vi "Queue Event Log.vi"(5 "System Data":T1 {"Converter Faults 2" format="%016b"; "Converter Alarms 2" format="%016b"; "Converter Faults 1" format="%016b"; "Converter Alarms 1" format="%016b"; "Solar Faults" format="%016b"; "ES Rack 10 Alarms" format="%016b"; "ES Rack 9 Alarms" format="%016b"; "ES Rack 8 Alarms" format="%016b"; "ES Rack 7 Alarms" format="%016b"; "ES Rack 6 Alarms" format="%016b"; "ES Rack 5 Alarms" format="%016b"; "ES Rack 4 Alarms" format="%016b"; "ES Rack 3 Alarms" format="%016b"; "ES Rack 2 Alarms" format="%016b"; "ES Rack 1 Alarms" format="%016b"; "ES System Alarms" format="%016b"; "System Faults" format="%016b"; "ES Rack 10 Faults" format="%016b"; "Es Rack 9 Faults" format="%016b"; "ES Rack 8 Faults" format="%016b"; "ES Rack 7 Faults" format="%016b"; "ES Rack 6 Faults" format="%016b"; "ES Rack 5 Faults" format="%016b"; "ES Rack 4 Faults" format="%016b"; "ES Rack 3 Faults" format="%016b"; "ES Rack 2 Faults" format="%016b"; "ES Rack 1 Faults" format="%016b"; "ES System Faults" format="%016b"; "System Status" format="%016b"; "Controller Faults" format="%016b"}, 7 "Connection Error":bool, 8 "Error In":errorcluster, 11 "Event Log Queue":refnum<queue>) -> (0 "Error Out":errorcluster)   [LabVIEW 2014]
uses:
  Controls/Modbus Status Interface Data MOD2.ctl
panel:
  in  "Gen East Faults":string
  in  "Gen West Faults":string
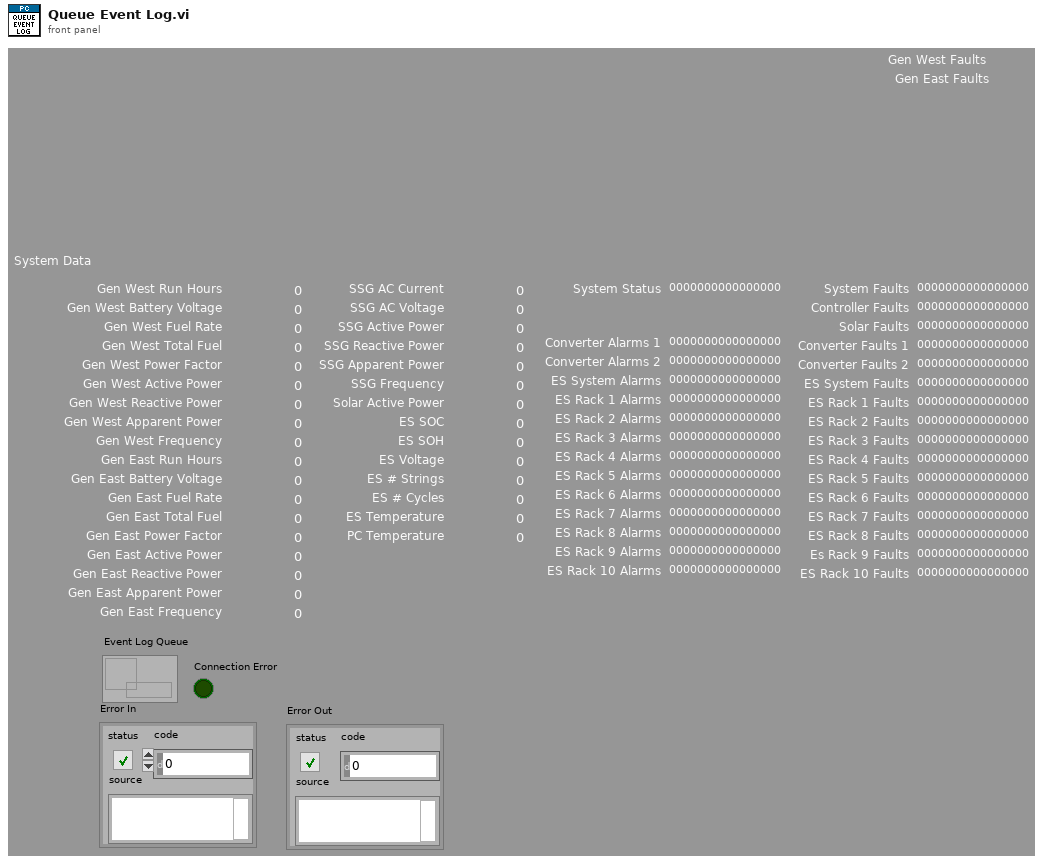
[diagram p1: front panel]
types:
  T1 = typedef "Modbus Status Interface Data MOD2.ctl" = cluster{"SSG AC Current":i16, "SSG AC Voltage":i16, "SSG Active Power":i16, "SSG Reactive Power":i16, "SSG Apparent Power":i16, "SSG Frequency":i16, "ES SOC":i16, "ES SOH":i16, "ES Voltage":i16, "ES # Strings":i16, "ES # Cycles":i16, "ES Temperature":i16, "PC Temperature":i16, "Solar Active Power":i16, "Gen West Run Hours":i16, "Gen West Battery Voltage":i16, "Gen West Fuel Rate":i16, "Gen West Total Fuel":i16, "Gen West Power Factor":i16, "Gen West Active Power":i16, "Gen West Reactive Power":i16, "Gen West Apparent Power":i16, "Gen West Frequency":i16, "Gen East Run Hours":i16, "Gen East Battery Voltage":i16, "Gen East Fuel Rate":i16, "Gen East Total Fuel":i16, "Gen East Power Factor":i16, "Gen East Active Power":i16, "Gen East Reactive Power":i16, "Gen East Apparent Power":i16, "Gen East Frequency":i16, "Converter Version":i16, "Controller Version":i16, "System Status":i16, "System Faults":i16, "Controller Faults":i16, "ES System Faults":i16, "ES System Alarms":i16, "Converter Faults 1":i16, "Converter Faults 2":i16, "Converter Alarms 1":i16, "Converter Alarms 2":i16, "Solar Faults":i16, "ES Rack 1 Faults":i16, "ES Rack 2 Faults":i16, "ES Rack 3 Faults":i16, "ES Rack 4 Faults":i16, "ES Rack 5 Faults":i16, "ES Rack 6 Faults":i16, "ES Rack 7 Faults":i16, "ES Rack 8 Faults":i16, "Es Rack 9 Faults":i16, "ES Rack 10 Faults":i16, "ES Rack 1 Alarms":i16, "ES Rack 2 Alarms":i16, "ES Rack 3 Alarms":i16, "ES Rack 4 Alarms":i16, "ES Rack 5 Alarms":i16, "ES Rack 6 Alarms":i16, "ES Rack 7 Alarms":i16, "ES Rack 8 Alarms":i16, "ES Rack 9 Alarms":i16, "ES Rack 10 Alarms":i16}
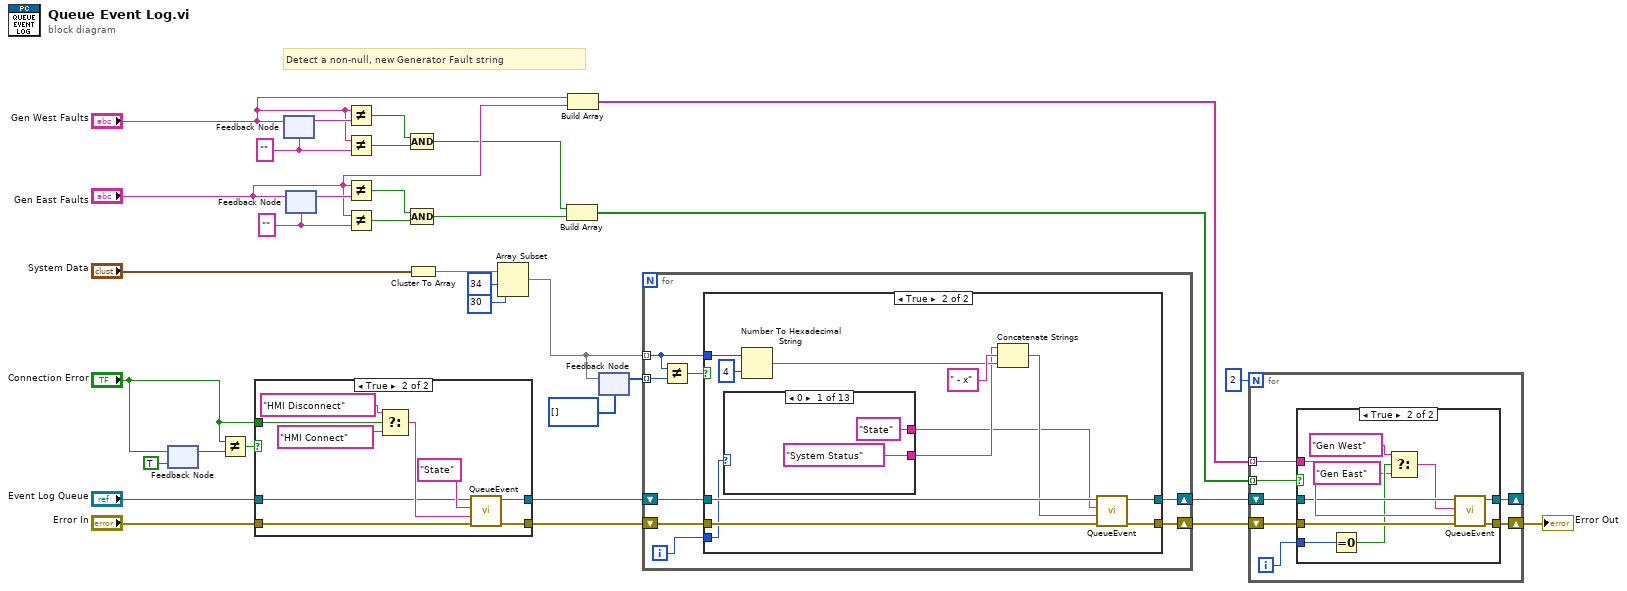
[diagram p0: block diagram]
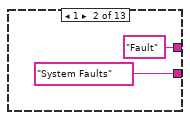
[diagram p4: hidden frame]
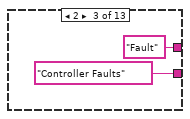
[diagram p5: hidden frame]
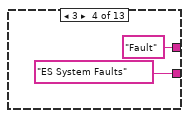
[diagram p6: hidden frame]
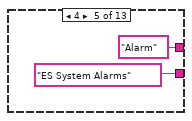
[diagram p7: hidden frame]
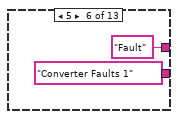
[diagram p8: hidden frame]
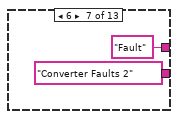
[diagram p9: hidden frame]
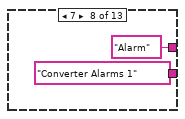
[diagram p10: hidden frame]
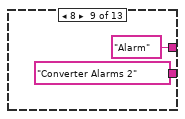
[diagram p11: hidden frame]
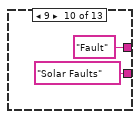
[diagram p12: hidden frame]
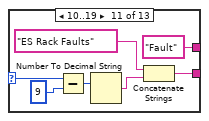
[diagram p13: hidden frame]
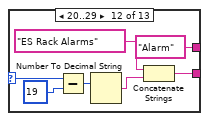
[diagram p14: hidden frame]
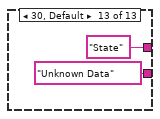
[diagram p15: hidden frame]
diagram:
  w9 = "" ("Gen West Faults")
  w7 = "" ("Gen West Faults")
  # "Detect a non-null, new Generator Fault string"
  n1 = feedback-in #1("Connection Error") -> ()
  n2 = feedback #1(TRUE ("Connection Error")) -> (w30:bool)
  n3 = Not Equal?(x="Connection Error", y=w30) -> (x != y?=w29:bool)
  n4 = case shown="True" w29 {
    tunnel: "Error In" -> [w35 w44]
    tunnel: [w35 w43] -> w22
    tunnel: "Event Log Queue" -> [w34 w38]
    tunnel: "Connection Error" -> [_ w37]
    tunnel: [w34 w36] -> w23
    frame False {
    }
    frame True {
      n5 = Select(t="HMI Disconnect" ("Event Name"), s=w37, f="HMI Connect") -> (s? t:f=w40:string)
      n6 = call "QueueEvent.vi"("Error In"=w44, "Event Description"=w40, "Event Name"="State", "Queue In"=w38) -> ("Error Out"=w43:errorcluster, "Queue Out"=w36:refnum<queue>)  [unwired: 6 in]
    }
  }
  n7 = feedback-in #2("Gen West Faults") -> ()
  n8 = feedback #2(w7) -> (w15:string)
  n9 = feedback #3(w9) -> (w16:string)
  n10 = feedback-in #3("Gen East Faults") -> ()
  n11 = Not Equal?(x="Gen West Faults", y=w15) -> (x != y?=w6:bool)
  n12 = Not Equal?(x="Gen West Faults", y=w7) -> (x != y?=w5:bool)
  n13 = Not Equal?(x="Gen East Faults", y=w16) -> (x != y?=w2:bool)
  n14 = Not Equal?(x="Gen East Faults", y=w9) -> (x != y?=w3:bool)
  n15 = Cluster To Array(cluster="System Data") -> (array=w26:i16[])
  n16 = Compound Arithmetic op=AND(w6, w5) -> (w4:bool)
  n17 = Compound Arithmetic op=AND(w2, w3) -> (w1:bool)
  n18 = Array Subset(array=w26, index=34, length=30) -> (w21:i16[])
  n19 = Build Array(w4, w1) -> (w14:bool[])
  n20 = Build Array("Gen West Faults", "Gen East Faults") -> (w13:string[])
  n21 = feedback-in #4(w21) -> ()
  n22 = feedback #4(i16[] []) -> (w20:i16[])
  n23 = for {
    tunnel: w21 -> [w46] mode=indexing
    shift-right: [w51] -> w11
    shift-left: w23 -> [w52]
    tunnel: w20 -> [w49] mode=indexing
    shift-right: [w45] -> w18
    shift-left: w22 -> [w50]
    i -> [w47]
    n24 = Not Equal?(x=w46, y=w49) -> (x != y?=w48:bool)
    n25 = case shown="True" w48 {
      tunnel: w52 -> [w54 w66]
      tunnel: [w54 w65] -> w51
      tunnel: w50 -> [w53 w64]
      tunnel: w47 -> [_ w57]
      tunnel: w46 -> [_ w63]
      tunnel: [w53 w58] -> w45
      frame False {
      }
      frame True {
        n26 = case shown="0" w57 {
          selector: w57 -> [_ _ _ _ _ _ _ _ _ _ w91 w98 _]
          tunnel: ["System Status" ("string") "System Faults" ("string") "Controller Faults" ("string") "ES System Faults" ("string") "ES System Alarms" ("string") "Converter Faults 1" ("string") "Converter Faults 2" ("string") "Converter Alarms 1" ("string") "Converter Alarms 2" ("string") "Solar Faults" ("string") w92 w99 "Unknown Data" ("string")] -> w56
          tunnel: ["State" ("Event Name") "Fault" ("Event Name") "Fault" ("Event Name") "Fault" ("Event Name") "Alarm" ("Event Name") "Fault" ("Event Name") "Fault" ("Event Name") "Alarm" ("Event Name") "Alarm" ("Event Name") "Fault" ("Event Name") "Fault" ("Event Name") "Alarm" ("Event Name") "State" ("Event Name")] -> w55
          frame 0 {
          }
          frame 1 {
          }
          frame 2 {
          }
          frame 3 {
          }
          frame 4 {
          }
          frame 5 {
          }
          frame 6 {
          }
          frame 7 {
          }
          frame 8 {
          }
          frame 9 {
          }
          frame 10..19 {
            n27 = Subtract(x=w91, y=9) -> (x-y=w89:i32)
            n28 = Number To Decimal String(number=w89) -> (decimal integer string=w88:string)  [unwired: 1 in]
            n29 = Concatenate Strings("ES Rack Faults" ("string"), w88) -> (w92:string)
          }
          frame 20..29 {
            n30 = Subtract(x=w98, y=19) -> (x-y=w96:i32)
            n31 = Number To Decimal String(number=w96) -> (decimal integer string=w95:string)  [unwired: 1 in]
            n32 = Concatenate Strings("ES Rack Alarms" ("string"), w95) -> (w99:string)
          }
          frame 30, Default {
          }
        }
        n33 = Number To Hexadecimal String(1:i16 4 ("width (-)"), 2:w63) -> (0:w59:string)
        n34 = Concatenate Strings(w56, " - x" ("string"), w59) -> (w61:string)
        n35 = call "QueueEvent.vi"("Error In"=w64, "Event Description"=w61, "Event Name"=w55, "Queue In"=w66) -> ("Error Out"=w58:errorcluster, "Queue Out"=w65:refnum<queue>)  [unwired: 6 in]
      }
    }
  }
  n36 = for {
    N: 2 -> [_]
    shift-right: [w108] -> w17
    shift-left: w18 -> [w109]
    tunnel: w14 -> [w107] mode=indexing
    tunnel: w13 -> [w106] mode=indexing
    shift-right: [w104] -> _
    shift-left: w11 -> [w105]
    i -> [w103]
    n37 = case shown="True" w107 {
      tunnel: w109 -> [w111 w121]
      tunnel: [w111 w120] -> w108
      tunnel: w106 -> [_ w119]
      tunnel: w105 -> [w110 w118]
      tunnel: [w110 w117] -> w104
      tunnel: w103 -> [_ w115]
      frame False {
      }
      frame True {
        n38 = Equal To 0?(x=w115) -> (x = 0?=w114:bool)
        n39 = Select(t="Gen West" ("Event Name"), s=w114, f="Gen East") -> (s? t:f=w112:string)
        n40 = call "QueueEvent.vi"("Error In"=w121, "Event Description"=w119, "Event Name"=w112, "Queue In"=w118) -> ("Error Out"=w120:errorcluster, "Queue Out"=w117:refnum<queue>)  [unwired: 6 in]
      }
    }
  }
  "Error Out" <- w17
